vi "girada_state_selection (SubVI).vi"(9 "Target":dbl[](array[numeric]), 10 "Robot in":refnum<class "Robot.lvclass">, 11 "Game in":refnum<class "Game.lvclass">) -> (3 "String":string)   [LabVIEW 2021]
uses:
  GiradaTypedefs/Control 3.ctl
  <vilib>/Analysis/NI_AALBase.lvlib
  Robot_class/Robot.lvclass
  C:/Users/IME/Desktop/Horie - VSS - SSL/SSL_AI/Object_class/Object.lvclass
  C:/Users/IME/Desktop/Horie - VSS - SSL/SSL_AI/Robot_class/Robot.lvclass
  Game_class/Game.lvclass
  Ball_class/Ball.lvclass
  <vilib>/Analysis/baseanly.llb/Real Dot Product.vi
panel:
  in  "Raio":dbl=123.0
  in  "Target 2":dbl[](array[numeric])
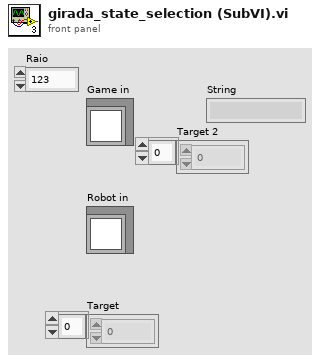
[diagram p1: front panel]
types:
  T1 = typedef "Control 3.ctl" = enum16{"go straight", "goig to the circule", "circulating the ball", "kicking"}
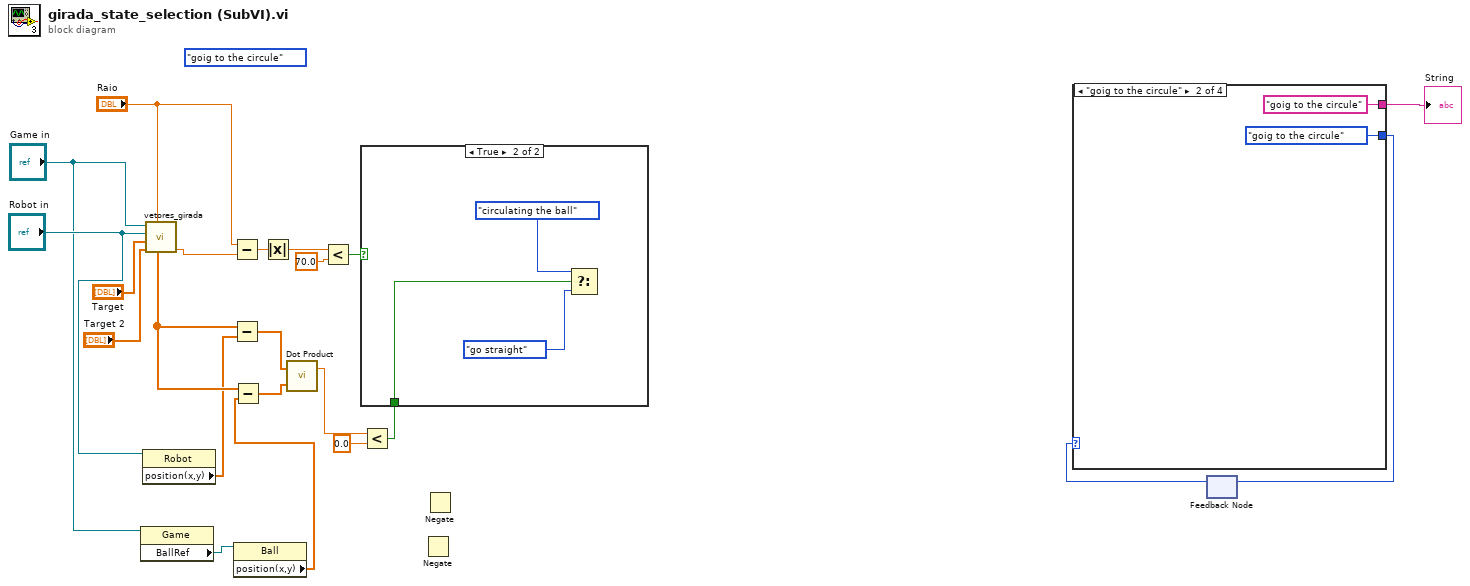
[diagram p0: block diagram]
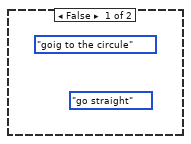
[diagram p2: hidden frame]
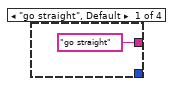
[diagram p3: hidden frame]
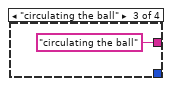
[diagram p4: hidden frame]
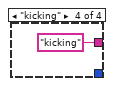
[diagram p5: hidden frame]
diagram:
  (unwired) Control_3."goig to the circule"
  n1 = property class="Game"(reference="Game in") -> ("BallRef"=w8:refnum<class "Ball.lvclass">)  [unwired: 1 in, 2 out]
  n2 = property class="Robot"(reference="Robot in") -> ("position(x,y)"=w6:dbl[])  [unwired: 1 in, 2 out]
  n3 = call "vetores_girada.vi"("Raio"="Raio", "Target"="Target 2", "Target 2"="Target", "Robot in"="Robot in", "Game in"="Game in") -> ("Norm RB"=w14:dbl, "robo position in circle location"=w11:dbl[])  [unwired: 5 out]
  n4 = Subtract(x="Raio", y=w14) -> (x-y=w12:dbl)
  n5 = Subtract(x=w11, y=w6) -> (x-y=w5:dbl[])
  n6 = property class="Ball"(reference=w8) -> ("position(x,y)"=w7:dbl[])  [unwired: 1 in, 2 out]
  n7 = Subtract(x=w11, y=w7) -> (x-y=w4:dbl[])
  n8 = Absolute Value(x=w12) -> (abs(x)=w19:dbl)
  n9 = call-poly <vilib>:"Dot Product.vi"("Y Vector"=w4, "X Vector"=w5) -> ("X * Y"=w3:dbl)  [unwired: 1 out]
  n10 = Less?(x=w19, y=70.0) -> (x < y?=w15:bool)
  n11 = Less?(x=w3, y=0.0) -> (x < y?=w1:bool)
  n12 = case shown="True" w15 {
    tunnel: w1 -> [_ w25]
    frame False {
      (unwired) Control_3."go straight"
      (unwired) Control_3."goig to the circule"
    }
    frame True {
      n13 = Select(t=Control_3."circulating the ball", s=w25, f=Control_3."go straight") -> ()  [unwired: 1 out]
    }
  }
  n14 = Negate() -> ()  [unwired: 1 in, 1 out]
  n15 = Negate() -> ()  [unwired: 1 in, 1 out]
  n16 = feedback #1() -> (w21:T1)  [unwired: 1 in]
  n17 = case shown="\"goig to the circule\"" w21 {
    tunnel: [_ Control_3."goig to the circule" _ _] -> w20
    tunnel: ["go straight" "goig to the circule" "circulating the ball" "kicking"] -> w22
    frame "go straight", Default {
    }
    frame "goig to the circule" {
    }
    frame "circulating the ball" {
    }
    frame "kicking" {
    }
  }
  "String" <- w22
  n18 = feedback-in #1(w20) -> ()
